vi "distance sensor.vi"() -> ()   [LabVIEW 2023]
doc: "Use this template to build a standard state machine design pattern. Each state executes code and determines which state to transition to. Contrast this design pattern with the User Interface Event Handler pattern, in which code executes in response to user actions. Contrast this design pattern also with the Queued Message Handler pattern, in which each message handling code can queue zero or more new messages.\nNote: This template does not contain the most recent programming guidelines recommended by National Instruments. For a complete, project-based implementation of the Standard State Machine pattern, use the Create Project dialog box instead of this template."
uses:
  <vilib>/userDefined/High Color/IMAQdx.ctl
  wasilistan.ctl
  <vilib>/vision/Image Controls.llb/IMAQ Image.ctl
  <vilib>/Instr/_visa.llb/VISA Configure Serial Port (Instr).vi
  <vilib>/regexp/Match Regular Expression.xnode
  <vilib>/vision/driver/NI_Vision_Acquisition_Software.lvlib
panel:
  out "Image":T1(plugin-control)
  in  "Kamerka 2":T2
  out "error out 2":errorcluster
  in  "Arduino":refnum<visa-resource-name>
  in  "symulator odleglosci":dbl
  out "Serial Settings:Number of Bytes at Serial Port":u32
  in  "STOP":bool
  out "Odleglosc":dbl
  out "read buffer":string
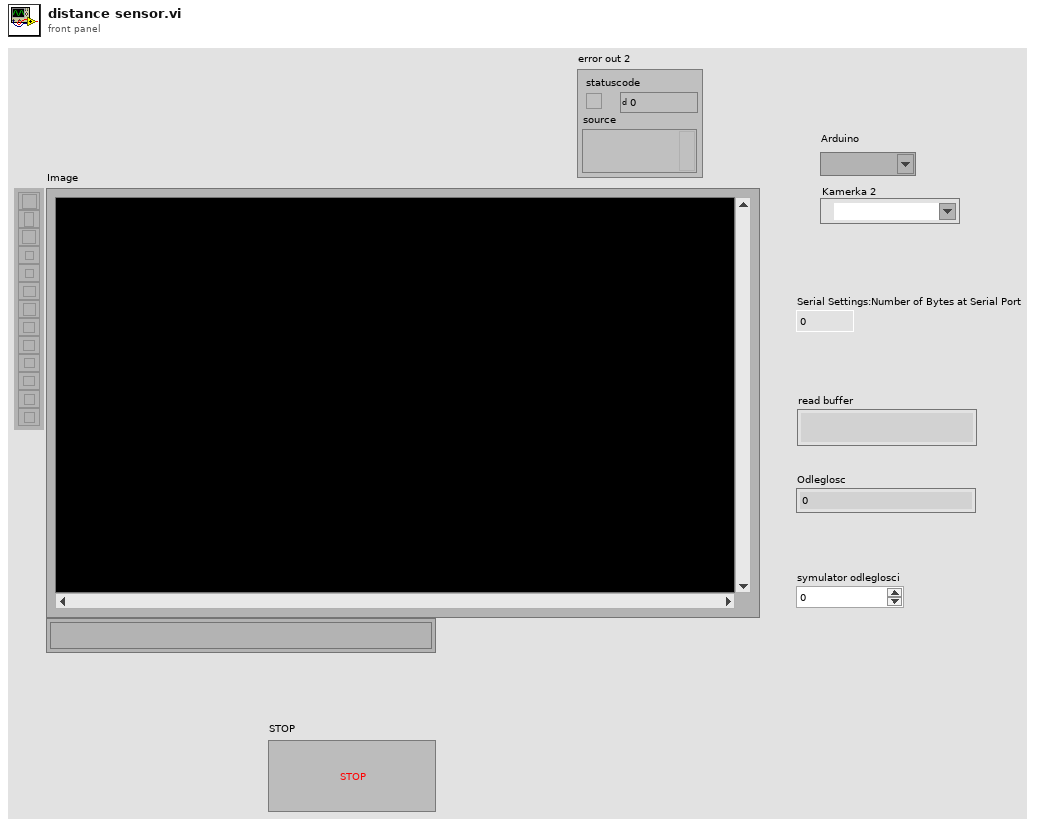
[diagram p1: front panel]
types:
  T1 = typedef "IMAQ Image.ctl" = refnum<image>
  T2 = typedef "IMAQdx.ctl" = refnum<k21>
  T3 = typedef "wasilistan.ctl" = enum16{"Initialize", "Czytaj", "Buzzer", "Kamera", "Stop"}
  T4 = typedef "Image Type" = u32
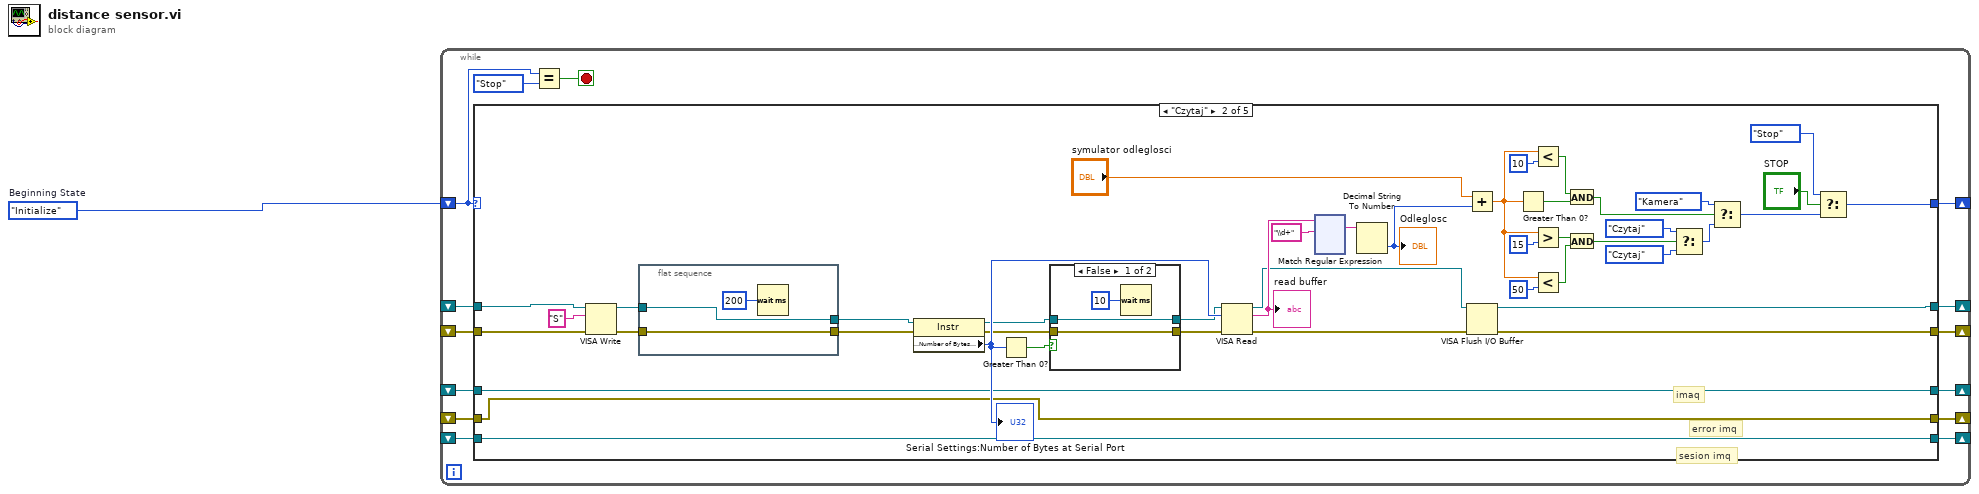
[diagram p0: block diagram]
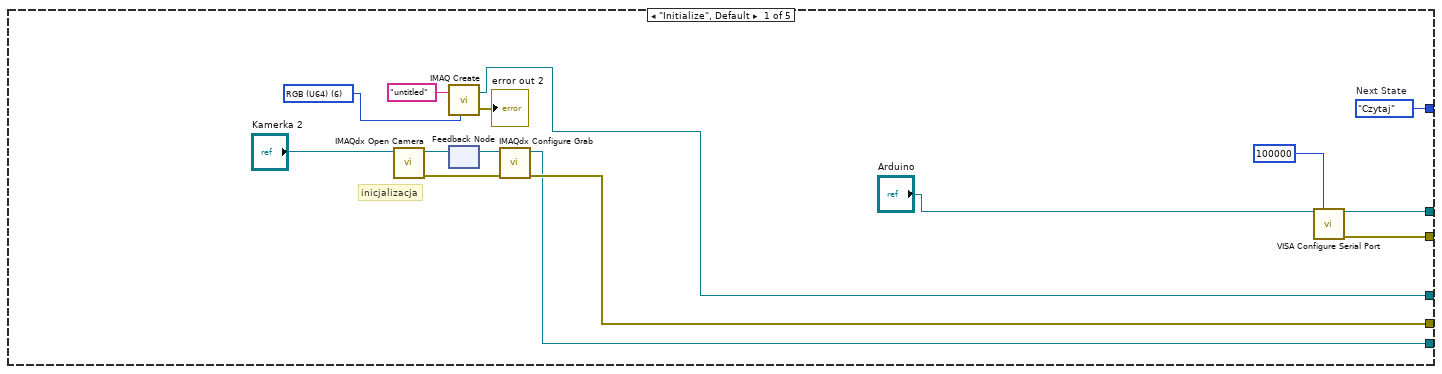
[diagram p2: hidden frame]
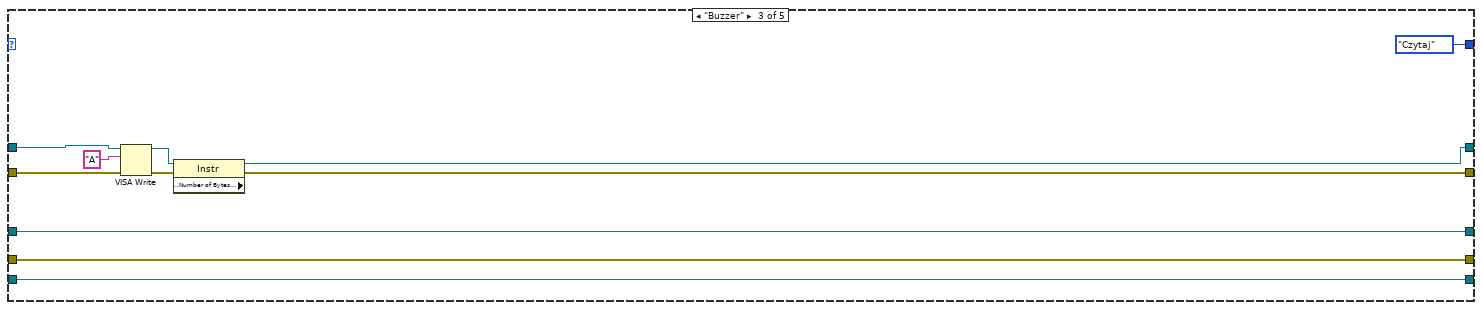
[diagram p4: hidden frame]
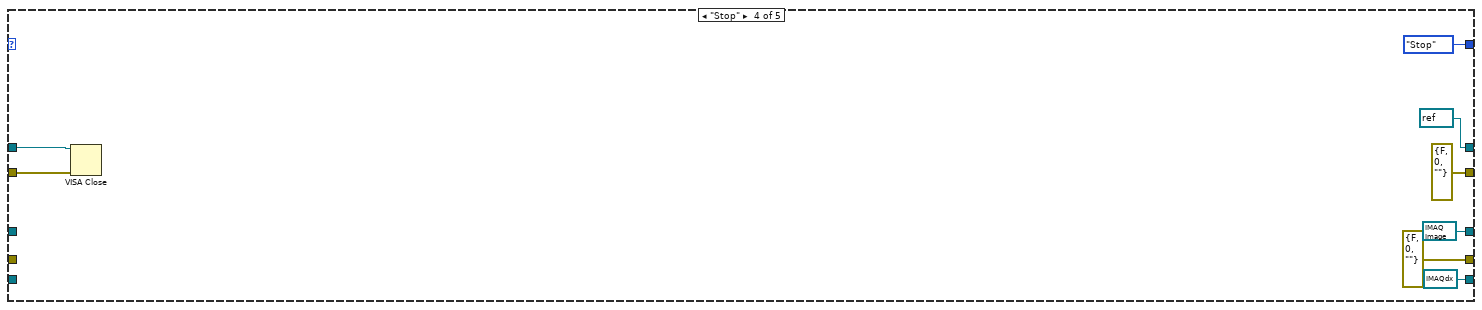
[diagram p5: hidden frame]
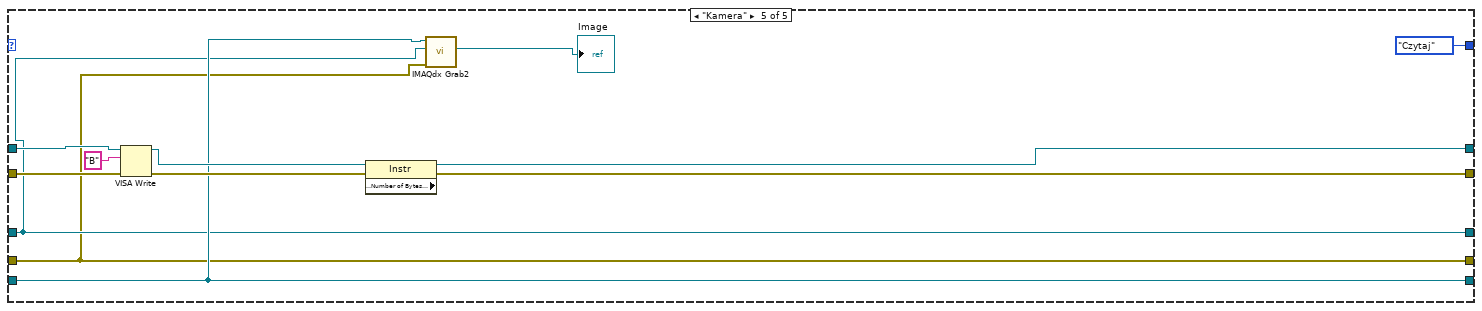
[diagram p6: hidden frame]
diagram:
  w1 = wasilistan."Initialize"  # Beginning State
  # "sesion imq"
  # "error imq"
  # "imaq"
  n1 = while {
    shift-right: [w13] -> _
    shift-left: w1 -> [w8]
    shift-right: [w12] -> _
    shift-left: _ -> [w10]
    shift-right: [w11] -> _
    shift-left: _ -> [w9]
    shift-right: [w7] -> _
    shift-left: _ -> [w2]
    shift-right: [w6] -> _
    shift-left: _ -> [w3]
    shift-right: [w5] -> _
    shift-left: _ -> [w4]
    stop <- w15 stop-if-true
    n2 = case shown="\"Czytaj\"" w8 {
      tunnel: [w30 w70 wasilistan."Czytaj" wasilistan."Stop" ("Next State") wasilistan."Czytaj"] -> w13
      tunnel: [w28 w41 w202 refnum<visa-resource-name> refnum ("VISA resource name out") w223] -> w12
      tunnel: [w27 w42 w203 errorcluster {"status"=FALSE, "code"=0, "source"=""} ("error constant") w222] -> w11
      tunnel: w10 -> [_ w69 w207 w216 w228]
      tunnel: w9 -> [_ w68 w208 w215 w227]
      tunnel: [w18 w31 w199 T1 refnum ("New Image") w219] -> w7
      tunnel: [w17 w32 w200 errorcluster {"status"=FALSE, "code"=0, "source"=""} ("error out") w218] -> w6
      tunnel: [w16 w33 w201 T2 refnum ("Session Out") w220] -> w5
      tunnel: w4 -> [_ w33 w201 _ w220]
      tunnel: w3 -> [_ w32 w200 _ w218]
      tunnel: w2 -> [_ w31 w199 _ w219]
      frame "Initialize", Default {
        w20 = T4 6 items=["Grayscale (U8)", "Grayscale (I16)", "Grayscale (SGL)", "Complex (CSG)", "RGB (U32)", "HSL (U32)", "RGB (U64)", "Grayscale (U16)"] ("Image Type")
        w30 = wasilistan."Czytaj"  # Next State
        # "inicjalizacja"
        n3 = call <vilib>:"IMAQdx Open Camera.vi"("Session In"="Kamerka 2") -> ("error out"=w23:errorcluster, "Session Out"=w25:T2)  [unwired: 9 in]
        n4 = call "IMAQ Create"("Image Name"="untitled", "Image Type"=w20) -> ("New Image"=w18:T1, "error out"=→"error out 2":errorcluster)  [unwired: 3 in]
        n5 = feedback #1() -> (w24:T2)  [unwired: 1 in]
        n6 = feedback-in #1(w25) -> ()
        n7 = call <vilib>:"IMAQdx Configure Grab.vi"("error in"=w23, "Session In"=w24) -> ("error out"=w17:errorcluster, "Session Out"=w16:T2)  [unwired: 8 in]
        n8 = call-poly "VISA Configure Serial Port"("VISA resource name"="Arduino", "timeout (10sec)"=u32 100000) -> ("VISA resource name out"=w28:refnum<visa-resource-name>, "error out"=w27:errorcluster)  [unwired: 12 in]
      }
      frame "Czytaj" {
        n9 = VISA Write(VISA resource name=w69, write buffer="S", error in (no error)=w68) -> (VISA resource name out=w66:refnum<visa-resource-name>, error out=w65:errorcluster)  [unwired: 1 out]
        n10 = flat-sequence {
          tunnel: [w81] -> w67
          tunnel: w66 -> [w81]
          tunnel: [w80] -> w64
          tunnel: w65 -> [w80]
          frame #0 {
            n11 = Wait (ms)(milliseconds to wait=u32 200) -> ()  [unwired: 1 out]
          }
        }
        n12 = property class="Instr"(reference=w67, error in=w64) -> (reference out=w47:refnum<visa-resource-name>, error out=w45:errorcluster, "Serial Settings:Number of Bytes at Serial Port"=w49:u32)
        "Serial Settings:Number of Bytes at Serial Port" <- w49
        n13 = Greater Than 0?(x=w49) -> (x > 0?=w48:bool)
        n14 = case shown="False" w48 {
          tunnel: [w76 w78] -> w46
          tunnel: w47 -> [w76 w78]
          tunnel: w45 -> [w75 w77]
          tunnel: [w75 w77] -> w44
          frame False {
            n15 = Wait (ms)(milliseconds to wait=u32 10) -> ()  [unwired: 1 out]
          }
          frame True {
          }
        }
        n16 = VISA Read(VISA resource name=w46, byte count=w49, error in (no error)=w44) -> (VISA resource name out=w40:refnum<visa-resource-name>, read buffer=w43:string, error out=w39:errorcluster)  [unwired: 1 out]
        "read buffer" <- w43
        n17 = xnode "Match Regular Expression"("input string"=w43, "regular expression"="\\d+") -> ("whole match"=w72:string)  [unwired: 4 in, 4 out]
        n18 = Decimal String To Number(string=w72) -> (number=w50:i32)  [unwired: 2 in, 1 out]
        "Odleglosc" <- w50
        n19 = Add(x="symulator odleglosci", y=w50) -> (x+y=w35:dbl)
        n20 = VISA Flush I/O Buffer(VISA resource name=w40, error in (no error)=w39) -> (VISA resource name out=w41:refnum<visa-resource-name>, error out=w42:errorcluster)  [unwired: 1 in]
        n21 = Greater Than 0?(x=w35) -> (x > 0?=w34:bool)
        n22 = Less?(x=w35, y=10) -> (x < y?=w36:bool)
        n23 = Greater?(x=w35, y=15) -> (0:w55:bool)
        n24 = Less?(x=w35, y=50) -> (x < y?=w54:bool)
        n25 = And(x=w36, y=w34) -> (x .and. y?=w37:bool)
        n26 = And(x=w55, y=w54) -> (x .and. y?=w57:bool)
        n27 = Select(t=wasilistan."Czytaj", s=w57, f=wasilistan."Czytaj") -> (s? t:f=w59:T3)
        n28 = Select(t=wasilistan."Kamera", s=w37, f=w59) -> (s? t:f=w61:T3)
        n29 = Select(t=wasilistan."Stop", s="STOP", f=w61) -> (s? t:f=w70:T3)
      }
      frame "Buzzer" {
        n30 = VISA Write(VISA resource name=w207, write buffer="A", error in (no error)=w208) -> (VISA resource name out=w205:refnum<visa-resource-name>, error out=w204:errorcluster)  [unwired: 1 out]
        n31 = property class="Instr" props=["Serial Settings:Number of Bytes at Serial Port"](reference=w205, error in=w204) -> (reference out=w202:refnum<visa-resource-name>, error out=w203:errorcluster)  [unwired: 1 out]
      }
      frame "Stop" {
        n32 = VISA Close(VISA resource name=w216, error in (no error)=w215) -> ()  [unwired: 1 out]
      }
      frame "Kamera" {
        n33 = VISA Write(VISA resource name=w228, write buffer="B", error in (no error)=w227) -> (VISA resource name out=w225:refnum<visa-resource-name>, error out=w224:errorcluster)  [unwired: 1 out]
        n34 = property class="Instr" props=["Serial Settings:Number of Bytes at Serial Port"](reference=w225, error in=w224) -> (reference out=w223:refnum<visa-resource-name>, error out=w222:errorcluster)  [unwired: 1 out]
        n35 = call <vilib>:"IMAQdx Grab2.vi"("error in"=w218, "Image In"=w219, "Session In"=w220) -> ("Image Out"=→"Image":T1)  [unwired: 5 in, 3 out]
      }
    }
    n36 = Equal?(x=w8, y=wasilistan."Stop" ("States")) -> (x = y?=w15:bool)
  }
